vi "Set Magnet.vi"(4 "Mode":T2, 6 "Axis":T1, 8 "error in (no error)":errorcluster, 9 "Target Rate (T/min)":dbl, 10 "Target Field (T)":dbl, 11 "Instrument.VRM in":refnum<class "Instrument.OxfordVRM.lvclass">) -> (0 "error out":errorcluster, 3 "Instrument.VRM out":refnum<class "Instrument.OxfordVRM.lvclass">)   [LabVIEW 2019, in "Instrument.OxfordVRM.lvclass"]
uses:
  Instrument.OxfordVRM.lvclass
  <userlib>/LevyLab/Levylab Instruments/Instrument Types/Cryostat/Typedefs/Magnet Mode--Enum.ctl
  <userlib>/LevyLab/Levylab Instruments/Instrument Types/Cryostat/Typedefs/Magnet Axis--Enum.ctl
  Typedefs/Instrument.VRM.Commands-enum.ctl
  Typedefs/Instrument.VRM.setMagnet-cluster.ctl
  Typedefs/VRM Targets--Cluster.ctl
  Typedefs/VRM Magnet Axis--Enum.ctl
  67c79f1b-78d1-46dd-8fbd-3891f861635a.vi
  67c79f1b-78d1-46dd-8fbd-3891f861635a.vi/d79cb1d2-5a09-4230-8614-1ed6ed9009d1.vi
  67c79f1b-78d1-46dd-8fbd-3891f861635a.vi/d79cb1d2-5a09-4230-8614-1ed6ed9009d1.vi/299041ac-6ae5-44b3-bb91-85af02e1dd41.vi
  67c79f1b-78d1-46dd-8fbd-3891f861635a.vi/d79cb1d2-5a09-4230-8614-1ed6ed9009d1.vi/c2bf7af8-bd7a-4f87-b164-4069121c5630.vi
  67c79f1b-78d1-46dd-8fbd-3891f861635a.vi/d79cb1d2-5a09-4230-8614-1ed6ed9009d1.vi/c2bf7af8-bd7a-4f87-b164-4069121c5630.vi/b0ccbbf6-060f-4f73-b067-726fc3845119.vi
  67c79f1b-78d1-46dd-8fbd-3891f861635a.vi/d79cb1d2-5a09-4230-8614-1ed6ed9009d1.vi/c2bf7af8-bd7a-4f87-b164-4069121c5630.vi/61d66cb0-7a77-4999-bb8d-6083244dc05b.vi
  <userlib>/LevyLab/Levylab Instruments/SMOs/RemoteControl/API/Remote Client.vi
  <vilib>/JDP Science/JSONtext/JSON text to Variant.vi
  <vilib>/JDP Science/JSONtext/LVClass Serializer/JSONtext LVClass Serializer.lvclass
  <userlib>/LevyLab/Levylab Instruments/Instrument Types/Cryostat/Instrument.Cryostat.lvclass
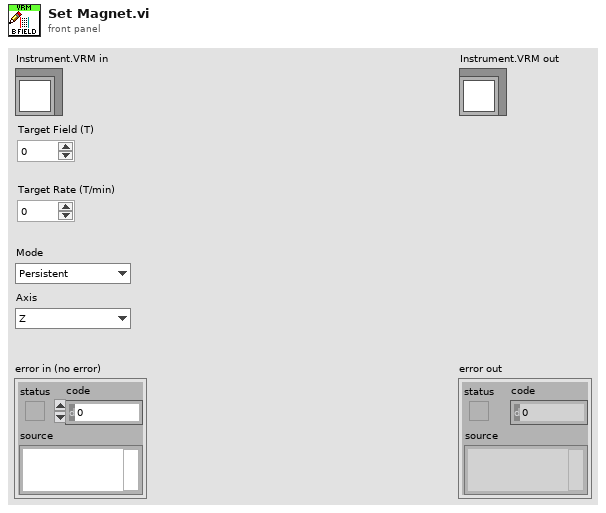
[diagram p1: front panel]
types:
  T1 = typedef "Instrument.Cryostat.lvclass/Magnet Axis--Enum.ctl" = enum16{"Z", "X", "Y"}
  T2 = typedef "Instrument.Cryostat.lvclass/Magnet Mode--Enum.ctl" = enum16{"Persistent", "Driven"}
  T3 = typedef "Instrument.OxfordVRM.lvclass/Instrument.VRM.setMagnet-cluster.ctl" = cluster{"Target":T4}
  T4 = typedef "Instrument.OxfordVRM.lvclass/VRM Targets--Cluster.ctl" = cluster{"Field (T)":dbl[], "Field Rate (T/min)":dbl, "Axis":T5}
  T5 = typedef "Instrument.OxfordVRM.lvclass/VRM Magnet Axis--Enum.ctl" = enum16{"Z", "X", "Y", "ALL"}
  T6 = typedef "Instrument.OxfordVRM.lvclass/Instrument.VRM.Commands-enum.ctl" = enum16{"setAction", "setTarget", "setMagnetField", "getStatus", "getTarget", "getMagnetField"}
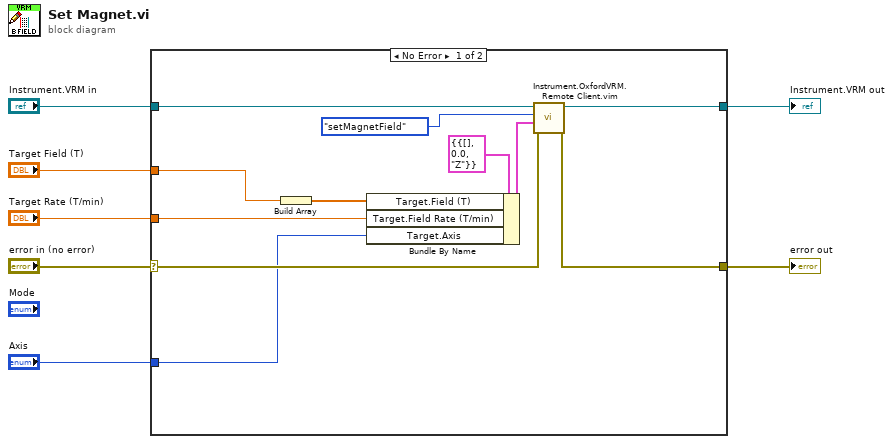
[diagram p0: block diagram]
diagram:
  n1 = case shown="No Error" "error in (no error)" {
    selector: "error in (no error)" -> [w16 w20]
    tunnel: "Target Rate (T/min)" -> [w18 _]
    tunnel: [w15 w20] -> w6
    tunnel: "Target Field (T)" -> [w9 _]
    tunnel: "Instrument.VRM in" -> [w14 w19]
    tunnel: [w17 w19] -> w3
    tunnel: "Axis" -> [w8 _]
    frame No Error {
      n2 = Build Array(w9) -> (w10:dbl[])
      n3 = Bundle By Name(cluster=T3 {"Target"={"Field (T)"=[], "Field Rate (T/min)"=0.0, "Axis"=enum."Z"}} ("output cluster"), "Target.Field (T)"=w10, "Target.Field Rate (T/min)"=w18, "Target.Axis"=w8) -> (w12:T3)
      n4 = call "Instrument.OxfordVRM.Remote Client.vim"("error in (no error)"=w16, "Data"=w12, "Commands"=Instrument.VRM.Commands-enum."setMagnetField", "Instrument.VRM in"=w14) -> ("error out"=w15:errorcluster, "Instrument.VRM out"=w17:refnum<class "Instrument.OxfordVRM.lvclass">)  [unwired: 5 in, 1 out]
    }
    frame Error {
    }
  }
  "Instrument.VRM out" <- w3
  "error out" <- w6
